vi "Pool.Get FIFO.vi"(11 "Pool in":refnum<class "Pool.lvclass">) -> (2 "FIFO":refnum<k33>, 3 "Pool out":refnum<class "Pool.lvclass">)   [LabVIEW 2017, in "DSF Core.lvlib" / "Pool.lvclass"]
uses:
  Pool.lvclass
  Pool.lvclass/Pool.ctl
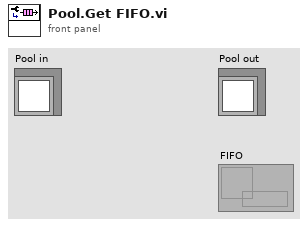
[diagram p1: front panel]
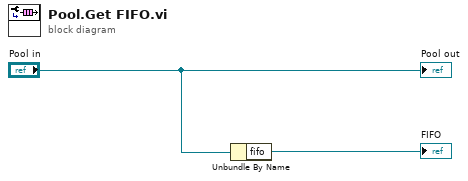
[diagram p0: block diagram]
diagram:
  n1 = Unbundle By Name("Pool in") -> ("fifo"=→"FIFO":refnum<k33>)
  "Pool out" <- "Pool in"
